vi "Trigger and Confirm.vi"(5 "Timestamp Channel (Confirm)":string, 6 "Timeout (s)":dbl=20.0 format="%#_13g", 7 "Trigger Channel":string, 8 "error in (no error)":errorcluster, 10 "Number of Triggers":i32=1, 11 "WorkspaceManager in":T1) -> (0 "error out":errorcluster, 3 "WorkspaceManager out":T1)   [LabVIEW 2023, in "Instrument Addon Common System Tests.lvclass"]
uses:
  Instrument Addon Common System Tests.lvclass
  <vilib>/NI VeriStand/Execution/Workspace/WorkspaceAPI.ctl
  NationalInstruments.VeriStand.ClientAPI
  <vilib>/NI VeriStand/Execution/Workspace/NI VeriStand - Get Single Channel Value.vi
  <vilib>/NI VeriStand/Execution/Workspace/NI VeriStand - Set Single Channel Value.vi
  <vilib>/NI VeriStand/Execution/Workspace/NI_VS Workspace ExecutionAPI.lvlib
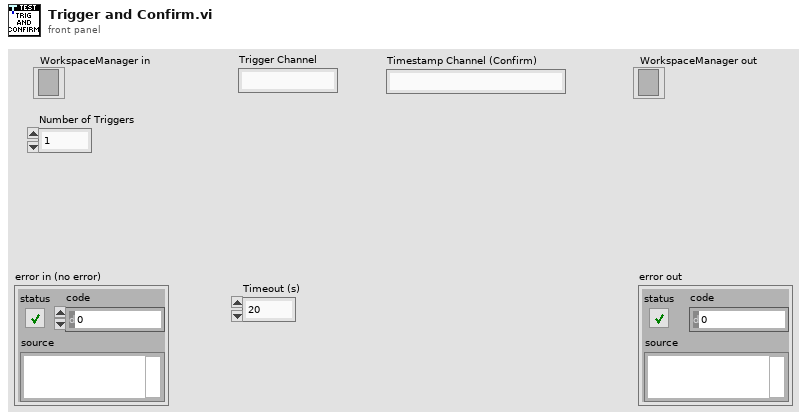
[diagram p1: front panel]
types:
  T1 = typedef "NI_VS Workspace ExecutionAPI.lvlib/WorkspaceAPI.ctl" = refnum<k24>
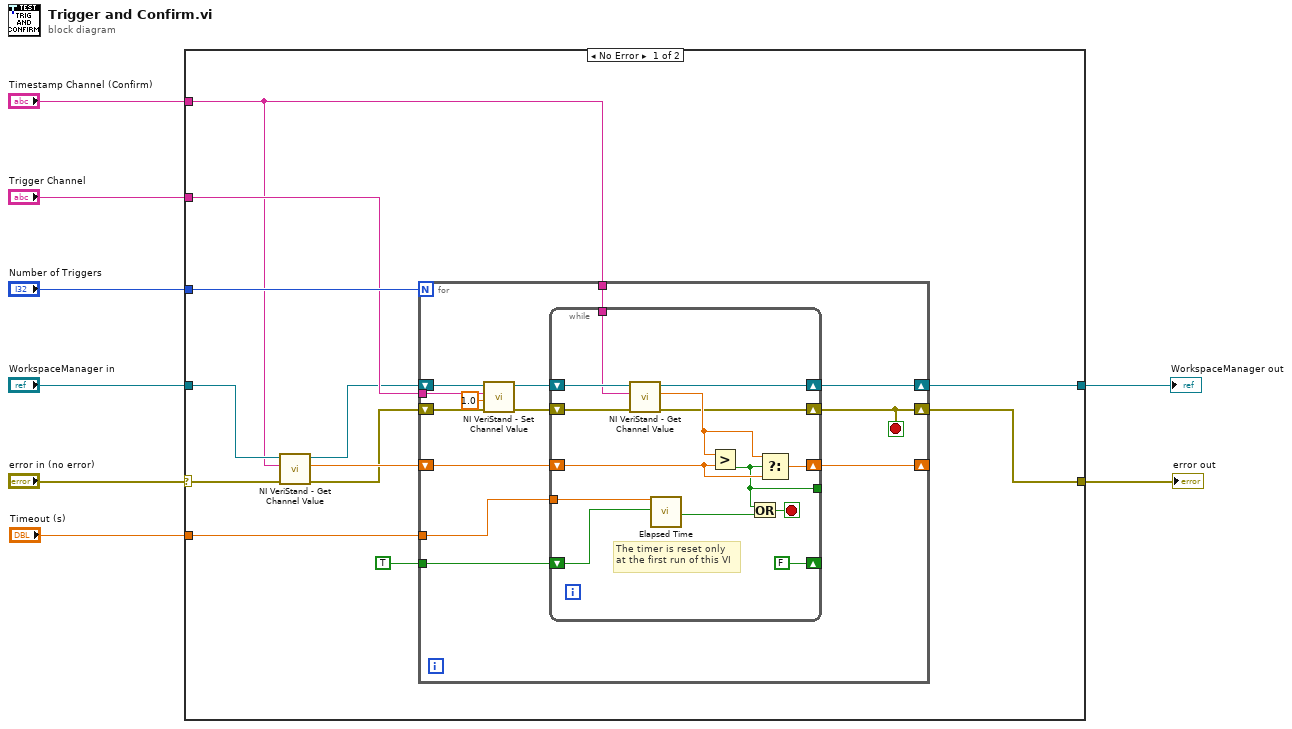
[diagram p0: block diagram]
diagram:
  n1 = case shown="No Error" "error in (no error)" {
    selector: "error in (no error)" -> [w11 w48]
    tunnel: "Number of Triggers" -> [w20 _]
    tunnel: [w19 w48] -> w7
    tunnel: "Trigger Channel" -> [w18 _]
    tunnel: "WorkspaceManager in" -> [w15 w49]
    tunnel: "Timestamp Channel (Confirm)" -> [w13 _]
    tunnel: [w12 w49] -> w3
    tunnel: "Timeout (s)" -> [w10 _]
    frame No Error {
      n2 = call-poly <vilib>:"NI VeriStand - Get Channel Value.vi"("error in (no error)"=w11, "Channel"=w13, "WorkspaceManager in"=w15) -> ("error out"=w16:errorcluster, "Value"=w17:dbl, "WorkspaceManager out"=w14:T1)  [unwired: 6 in]
      n3 = for {
        N: w20 -> [_]
        tunnel: w18 -> [w33]
        shift-right: [w24] -> w19
        shift-left: w16 -> [w28]
        shift-right: [w26] -> w12
        shift-left: w14 -> [w31]
        tunnel: w13 -> [w27]
        shift-right: [w25] -> _
        shift-left: w17 -> [w30]
        tunnel: w10 -> [w22]
        tunnel: TRUE ("Reset") -> [w21]
        stop <- w24 stop-if-true
        n4 = call-poly <vilib>:"NI VeriStand - Set Channel Value.vi"("error in (no error)"=w28, "Value"=1.0, "Channel"=w33, "WorkspaceManager in"=w31) -> ("error out"=w29:errorcluster, "WorkspaceManager out"=w32:T1)  [unwired: 6 in]
        n5 = while {
          shift-right: [w45] -> w26
          shift-left: w32 -> [w47]
          shift-right: [w37] -> w24
          shift-left: w29 -> [w46]
          shift-right: [w44] -> w25
          shift-left: w30 -> [w39]
          tunnel: [w38] -> _
          tunnel: w27 -> [w41]
          tunnel: w22 -> [w36]
          shift-right: [FALSE] -> _
          shift-left: w21 -> [w35]
          stop <- w42 stop-if-true
          # "The timer is reset only\nat the first run of this VI"
          n6 = call-poly <vilib>:"NI VeriStand - Get Channel Value.vi"("error in (no error)"=w46, "Channel"=w41, "WorkspaceManager in"=w47) -> ("error out"=w37:errorcluster, "Value"=w40:dbl, "WorkspaceManager out"=w45:T1)  [unwired: 6 in]
          n7 = call "Elapsed Time"("Time Target (s)"=w36, "Reset"=w35) -> ("Time has Elapsed"=w43:bool)  [unwired: 10 in, 7 out]
          n8 = Greater?(x=w40, y=w39) -> (0:w38:bool)
          n9 = Or(x=w38, y=w43) -> (x .or. y?=w42:bool)
          n10 = Select(t=w40, s=w38, f=w39) -> (s? t:f=w44:dbl)
        }
      }
    }
    frame Error {
    }
  }
  "error out" <- w7
  "WorkspaceManager out" <- w3
